vi "Close DO.vi"(8 "error in (no error)":errorcluster, 10 "data":bool[](array[boolean]), 11 "PXIe 6363 in":refnum<class "PXIe 6363.lvclass">) -> (0 "error out":errorcluster, 3 "PXIe 6363 out":refnum<class "PXIe 6363.lvclass">)   [LabVIEW 2021, in "DAQ Hardware.lvlib" / "PXIe 6363.lvclass"]
uses:
  PXIe 6363.lvclass
  <vilib>/DAQmx/write.llb/DAQmx Write (Digital 1D Bool NChan 1Samp 1Line).vi
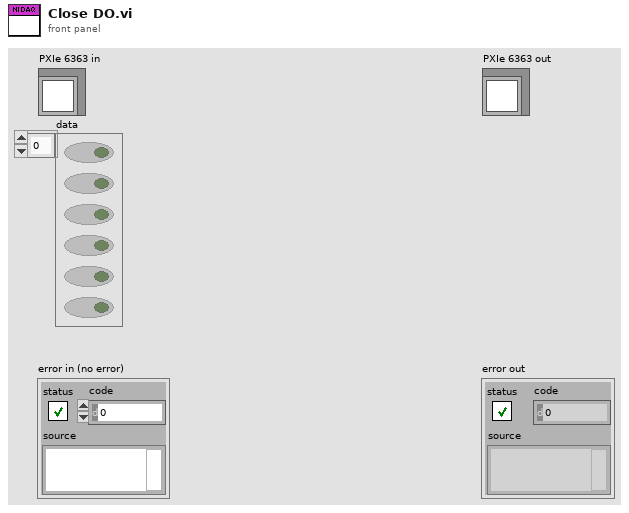
[diagram p1: front panel]
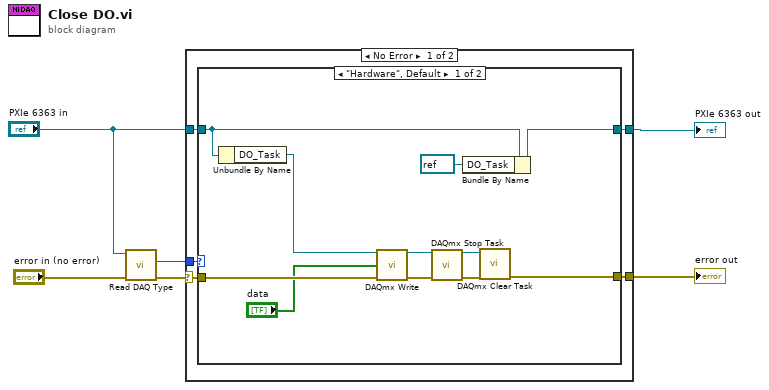
[diagram p0: block diagram]
diagram:
  n1 = call-dynamic "Read DAQ Type.vi"("error in (no error)"="error in (no error)", "PXIe 6363 in"="PXIe 6363 in") -> ("error out"=w5:errorcluster, "DAQ Type"=w4:enum16{"Hardware", "Simulation"})  [unwired: 7 in, 1 out]
  n2 = case shown="No Error" w5 {
    selector: w5 -> [w9 w25]
    tunnel: w4 -> [w11 _]
    tunnel: "PXIe 6363 in" -> [w10 w26]
    tunnel: [w8 w25] -> w2
    tunnel: [w7 w26] -> w1
    frame No Error {
      n3 = case shown="\"Hardware\", Default" w11 {
        tunnel: w10 -> [w19 w24]
        tunnel: w9 -> [w22 w23]
        tunnel: [w20 w23] -> w8
        tunnel: [w18 w24] -> w7
        frame "Hardware", Default {
          n4 = Unbundle By Name(w19) -> ("DO_Task"=w21:refnum<k21>)
          n5 = call-poly <vilib>:"DAQmx Write.vi"("task/channels in"=w21, "data"="data", "error in"=w22) -> ("task out"=w12:refnum<k21>, "error out"=w13:errorcluster)  [unwired: 10 in, 1 out]
          n6 = call <vilib>:"DAQmx Stop Task.vi"("task/channels in"=w12, "error in"=w13) -> ("task out"=w15:refnum<k21>, "error out"=w14:errorcluster)  [unwired: 12 in]
          n7 = Bundle By Name(cluster=w19, "DO_Task"=refnum<k21> refnum ("DO Task")) -> (w18:refnum<class "PXIe 6363.lvclass">)
          n8 = call <vilib>:"DAQmx Clear Task.vi"("task in"=w15, "error in"=w14) -> ("error out"=w20:errorcluster)  [unwired: 13 in]
        }
        frame "Simulation" {
        }
      }
    }
    frame Error {
    }
  }
  "error out" <- w2
  "PXIe 6363 out" <- w1
